vi "nD Line Search.vi"(0 "J":dbl[][](array[numeric]) format="%.2f", 5 "result":dbl[][](array[numeric]) format="%.2f", 6 "list of variables":i32[](array[numeric])=[0, 0], 7 "table":i32[][][](array[numeric]), 8 "TOLX":dbl=1e-07 format="%.2e", 9 "alpha":dbl=0.0001 format="%.2e", 10 "P":dbl[](array[numeric]) format="%.2f", 11 "X":dbl[](array[numeric]) format="%.2f") -> (2 "index":u32, 3 "X (new)":dbl[](array[numeric]) format="%.2f")   [LabVIEW 2020, in "NI_Gmath.lvlib"]
uses:
  NI_Gmath.lvlib
  NI_AALBase.lvlib
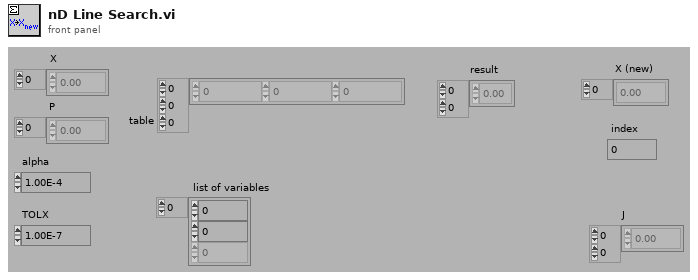
[diagram p1: front panel]
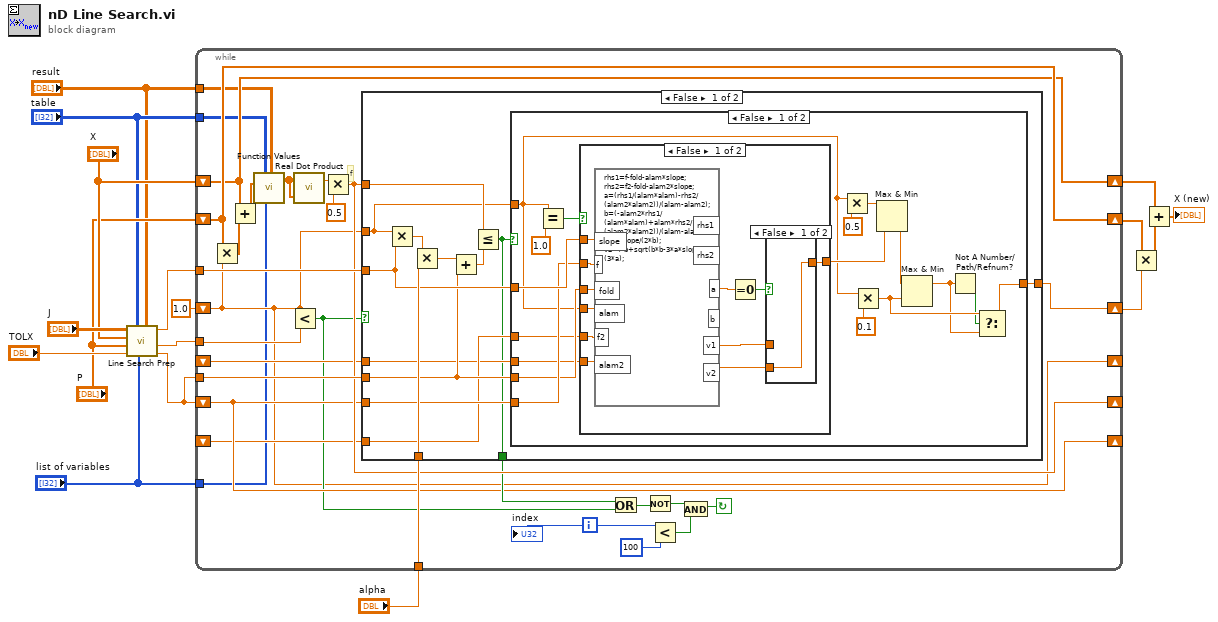
[diagram p0: block diagram]
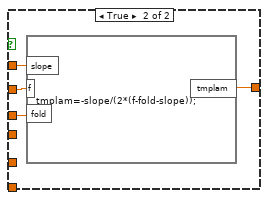
[diagram p3: hidden frame]
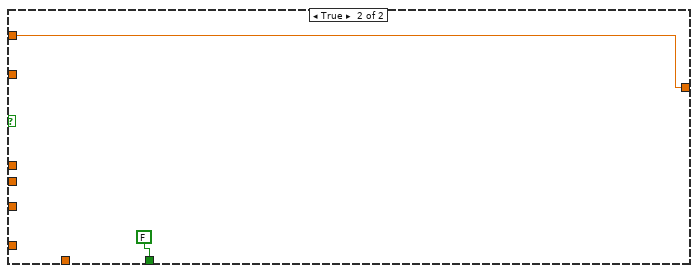
[diagram p5: hidden frame]
diagram:
  n1 = call "Line Search Prep.vi"("result"="result", "list of variables"="list of variables", "table"="table", "TOLX"="TOLX", "P"="P", "X"="X", "J"="J") -> ("F(X)*F(X)"=w12:dbl, "tolerance"=w14:dbl, "X * Y"=w13:dbl)  [unwired: 2 in]
  n2 = while {
    tunnel: w12 -> [w41]
    tunnel: w13 -> [w42]
    tunnel: "alpha" -> [w43]
    tunnel: w14 -> [w44]
    shift-left: _ -> [w34]
    shift-right: [w35] -> _
    shift-left: w12 -> [w35]
    shift-right: [w37] -> _
    shift-left: _ -> [w33]
    shift-right: [w27] -> _
    shift-left: 1.0 -> [w27]
    shift-right: [w26] -> w10
    shift-left: "P" -> [w32]
    shift-right: [w32] -> w9
    shift-left: "X" -> [w31]
    shift-right: [w31] -> w11
    tunnel: "result" -> [w20]
    tunnel: "table" -> [w19]
    tunnel: "list of variables" -> [w18]
    i -> [w30]
    stop <- w21 continue-if-true
    # "f"
    n3 = Multiply(x=w32, y=w27) -> (x*y=w45:dbl[])
    n4 = Add(x=w31, y=w45) -> (x+y=w25:dbl[])
    n5 = call "Function Values.vi"("result"=w20, "list of variables"=w18, "table"=w19, "X"=w25) -> ("F(X)"=w40:dbl[])  [unwired: 7 in]
    n6 = Less?(x=w27, y=w44) -> (x < y?=w29:bool)
    n7 = call "Real Dot Product.vi"("Y Vector"=w40, "X Vector"=w40) -> ("X * Y"=w39:dbl)  [unwired: 1 out]
    n8 = Multiply(x=w39, y=0.5) -> (x*y=w37:dbl)
    n9 = case shown="False" w29 {
      tunnel: w43 -> [w58 _]
      tunnel: w27 -> [w53 w94]
      tunnel: w42 -> [w51 _]
      tunnel: w41 -> [w49 _]
      tunnel: w37 -> [w54 _]
      tunnel: [w46 FALSE] -> w36
      tunnel: [w52 w94] -> w26
      tunnel: w35 -> [w50 _]
      tunnel: w34 -> [w48 _]
      tunnel: w33 -> [w47 _]
      frame False {
        n10 = Multiply(x=w53, y=w51) -> (x*y=w57:dbl)
        n11 = Multiply(x=w57, y=w58) -> (x*y=w56:dbl)
        n12 = Add(x=w56, y=w49) -> (x+y=w55:dbl)
        n13 = Less Or Equal?(x=w54, y=w55) -> (x <= y?=w46:bool)
        n14 = case shown="False" w46 {
          tunnel: w53 -> [w65 w93]
          tunnel: [w60 w93] -> w52
          tunnel: w51 -> [w68 _]
          tunnel: w50 -> [w67 _]
          tunnel: w49 -> [w66 _]
          tunnel: w48 -> [w64 _]
          tunnel: w47 -> [w63 _]
          frame False {
            n15 = Equal?(x=w65, y=1.0) -> (x = y?=w74:bool)
            n16 = case shown="False" w74 {
              tunnel: [w77 w92] -> w71
              tunnel: w68 -> [w86 w91]
              tunnel: w67 -> [w85 w90]
              tunnel: w66 -> [w84 w89]
              tunnel: w65 -> [w83 _]
              tunnel: w64 -> [w82 _]
              tunnel: w63 -> [w81 _]
              frame False {
                n17 = formula code="rhs1=f-fold-alam*slope;\nrhs2=f2-fold-alam2*slope;\na=(rhs1/(alam*alam)-rhs2/(alam2*alam2))/(alam-alam2);\nb=(-alam2*rhs1/(alam*alam)+alam*rhs2/(alam2*alam2))/(alam-alam2);\nv1=-slope/(2*b);\nv2=(-b+sqrt(b*b-3*a*slope))/(3*a);"("slope"=w86, "f"=w85, "fold"=w84, "alam"=w83, "f2"=w82, "alam2"=w81) -> ("a"=w80:dbl, "v1"=w78:dbl, "v2"=w76:dbl)  [unwired: 3 out]
                n18 = Equal To 0?(x=w80) -> (x = 0?=w79:bool)
                n19 = case shown="False" w79 {
                  tunnel: w78 -> [_ w88]
                  tunnel: [w87 w88] -> w77
                  tunnel: w76 -> [w87 _]
                  frame False {
                  }
                  frame True {
                  }
                }
              }
              frame True {
                n20 = formula code="tmplam=-slope/(2*(f-fold-slope));"("slope"=w91, "f"=w90, "fold"=w89) -> ("tmplam"=w92:dbl)
              }
            }
            n21 = Multiply(x=w65, y=0.5) -> (x*y=w72:dbl)
            n22 = Multiply(x=w65, y=0.1) -> (x*y=w62:dbl)
            n23 = Max & Min(x=w72, y=w71) -> (min(x,y)=w69:dbl)  [unwired: 1 out]
            n24 = Max & Min(x=w69, y=w62) -> (max(x,y)=w61:dbl)  [unwired: 1 out]
            n25 = Not A Number/Path/Refnum?(number/path/refnum=w61) -> (NaN/Path/Refnum?=w59:bool)
            n26 = Select(t=w62, s=w59, f=w61) -> (s? t:f=w60:dbl)
          }
          frame True {
          }
        }
      }
      frame True {
      }
    }
    n27 = Or(x=w36, y=w29) -> (x .or. y?=w28:bool)
    n28 = Not(x=w28) -> (.not. x?=w22:bool)
    n29 = Less?(x=w30, y=100) -> (x < y?=w23:bool)
    n30 = And(x=w22, y=w23) -> (x .and. y?=w21:bool)
    "index" <- w30
  }
  n31 = Multiply(x=w9, y=w10) -> (x*y=w8:dbl[])
  n32 = Add(x=w11, y=w8) -> (x+y=→"X (new)":dbl[])
